vi "Lock-in Default parameters.vi"(8 "error in (no error)":errorcluster, 11 "Handle in":T1 {"Handle" format="0x%08x"; "Conn" format="0x%08x"}) -> (0 "error out":errorcluster, 2 "zi_node":T2, 3 "Handle out":T1 {"Handle" format="0x%08x"; "Conn" format="0x%08x"})   [LabVIEW 2016]
uses:
  Controls/zi_node.ctl
  <instrlib>/Zurich Instruments LabOne/Public/ziTypeHandle.ctl
  <instrlib>/Zurich Instruments LabOne/Public/Configure/ziSetValueDoubleArray.vi
  <instrlib>/Zurich Instruments LabOne/Zurich Instruments LabOne.lvlib
panel:
  in  "zi_node":T2
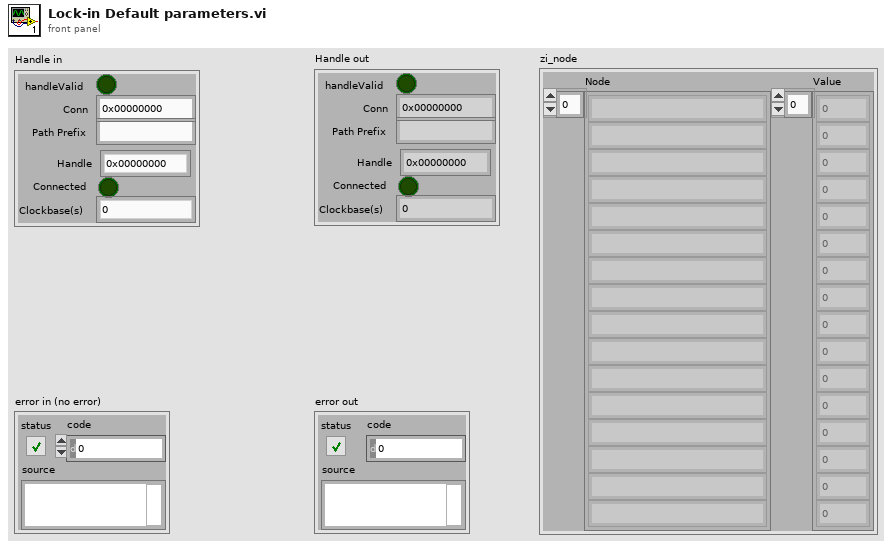
[diagram p1: front panel]
types:
  T1 = typedef "Zurich Instruments LabOne.lvlib/ziTypeHandle.ctl" = cluster{"handleValid":bool, "Conn":u64, "Path Prefix":string, "Handle":u64, "Connected":bool, "Clockbase(s)":dbl}
  T2 = typedef "zi_node.ctl" = cluster{"Node":string[], "Value":dbl[]}
  T3 = cluster{"Paths":string[], "Value":dbl[], "Comments":string[]}
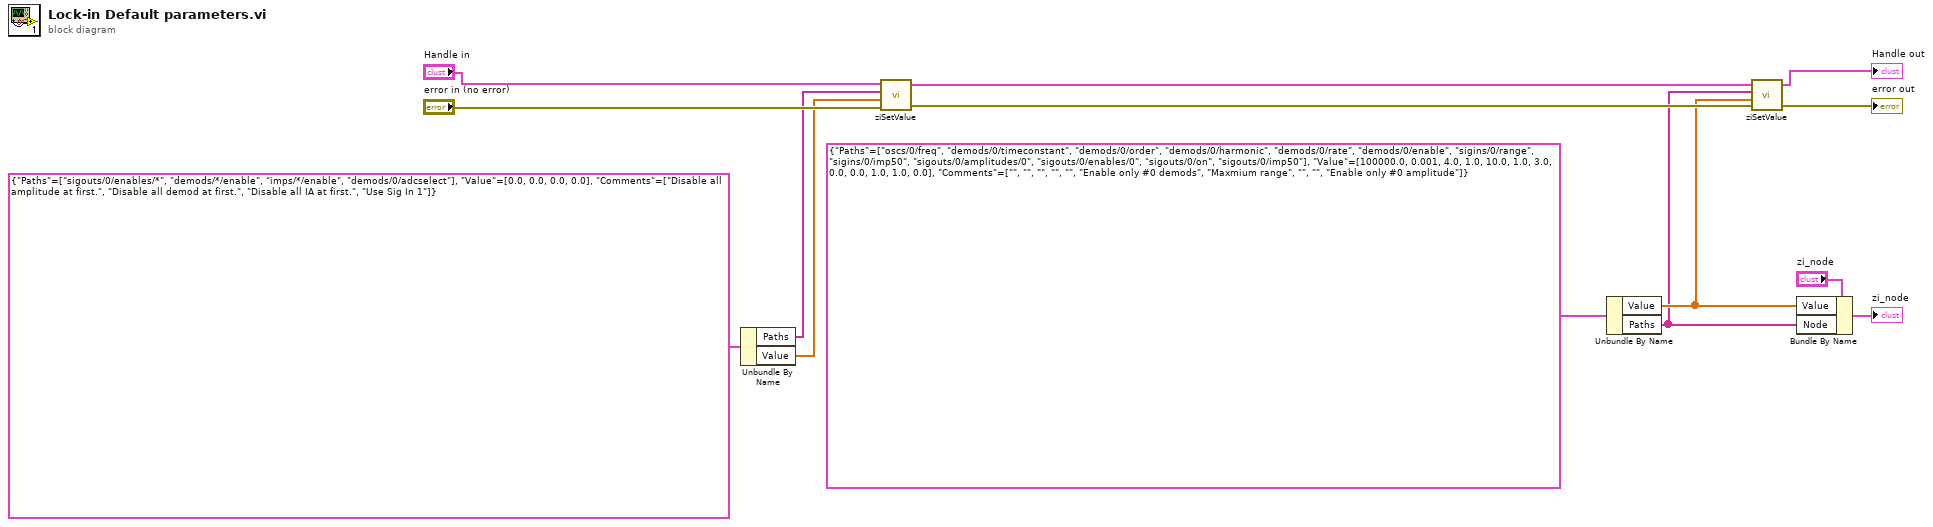
[diagram p0: block diagram]
diagram:
  n1 = Unbundle By Name(T3 {"Paths"=["sigouts/0/enables/*", "demods/*/enable", "imps/*/enable", "demods/0/adcselect"], "Value"=[0.0, 0.0, 0.0, 0.0], "Comments"=["Disable all amplitude at first.", "Disable all demod at first.", "Disable all IA at first.", "Use Sig In 1"]}) -> ("Paths"=w6:string[], "Value"=w5:dbl[])
  n2 = call-poly <instrlib>:"ziSetValue.vi"("Error In"="error in (no error)", "Values"=w5, "Paths"=w6, "Handle In"="Handle in") -> ("Error Out"=w10:errorcluster, "Handle Out"=w9:T1)  [unwired: 1 in]
  n3 = Unbundle By Name(T3 {"Paths"=["oscs/0/freq", "demods/0/timeconstant", "demods/0/order", "demods/0/harmonic", "demods/0/rate", "demods/0/enable", "sigins/0/range", "sigins/0/imp50", "sigouts/0/amplitudes/0", "sigouts/0/enables/0", "sigouts/0/on", "sigouts/0/imp50"], "Value"=[100000.0, 0.001, 4.0, 1.0, 10.0, 1.0, 3.0, 0.0, 0.0, 1.0, 1.0, 0.0], "Comments"=["", "", "", "", "", "Enable only #0 demods", "Maxmium range", "", "", "Enable only #0 amplitude"]}) -> ("Value"=w2:dbl[], "Paths"=w1:string[])
  n4 = call-poly <instrlib>:"ziSetValue.vi"("Error In"=w10, "Values"=w2, "Paths"=w1, "Handle In"=w9) -> ("Error Out"=→"error out":errorcluster, "Handle Out"=→"Handle out":T1)  [unwired: 1 in]
  n5 = Bundle By Name(cluster="zi_node", "Value"=w2, "Node"=w1) -> (→"zi_node":T2)
